vi "oax_gsExtract Order Waveform.vi"() -> ()   [LabVIEW 2017]
doc: "This VI provides Gabor order track, which can extract order from sound / vibration signal and playback on multimedia devices. This VI also provides access to Order Map.vi, which displays spectral maps, in menu bar window>> Show Order Map."
uses:
  <vilib>/addons/Sound and Vibration/Order Analysis/Ref Gabor Order Tracking/window information.ctl
  <vilib>/Analysis/1siggen.llb/Ramp Pattern by Samples.vi
  <vilib>/addons/Sound and Vibration/Order Analysis/Example Support/Demo VI/subVIs/oax_gsglobal variable.vi
  <vilib>/addons/Sound and Vibration/Order Analysis/Gabor Order Tracking/SoundVib_Gabor.lvlib
  <vilib>/Analysis/NI_AALBase.lvlib
panel:
  out "Selected File":string
  in  "Load Data":bool
  in  "user data path":path
  in  "Select Data":i32(listbox)
  in  "STOP":bool
  in  "track 3":bool
  in  "track 2":bool
  out "Speed at\nCursor (RPM)":dbl
  out "Time at\nCursor (sec)":dbl format="%.2f"
  in  "last path":path
  in  "unit":u16(ring) items=["Order", "Hz"]
  out "window information":T1={"window type"=3, "window length"=1} {"window type" items=["None"=0, "Hanning"=1, "Hamming"=2, "Blackman-Harris"=3, "Exact Blackman"=4, "Blackman"=5, "Flat Top"=6, "4 Term B-Harris"=7, "7 Term B-Harris"=8, "Low Sidelobe"=9, "Gaussian"=62]; "window length" min=0}
  out "TF Plot":u8[][](graph) caption="Time-Frequency Plot"
  out "Cursor Position":cluster{"Cursor X":dbl, "Cursor Y":dbl}={"Cursor X"=347.3140311804009, "Cursor Y"=0.0} {"Cursor Y" format="%.2f"; "Cursor X" format="%.2f"}
  in  "Play Sound":T2(ring)
  in  "Order List":i32[](listbox)
  out "Spectrum":cluster{dbl[], "X":dbl[]}(graph)
  out "mask":bool[][](array[boolean])
  in  "Bandwidth":dbl(slide)=0.5 min=0.0 scale=0.0..1.0 scale format="%.2f"
  in  "track":bool
  out "X":dbl[](array[numeric]) format="%.2f"
  in  "Selected Order":dbl min=0.0 step=0.10000000149011612 format="%.1f"
  out "Window \nLength":i32
  out "Status":string="Waiting..."
  out "Sample \nRate (Hz)":dbl
  out "S&V plot":dbl[][](graph)
  # "Narrow"
  # "Wide"
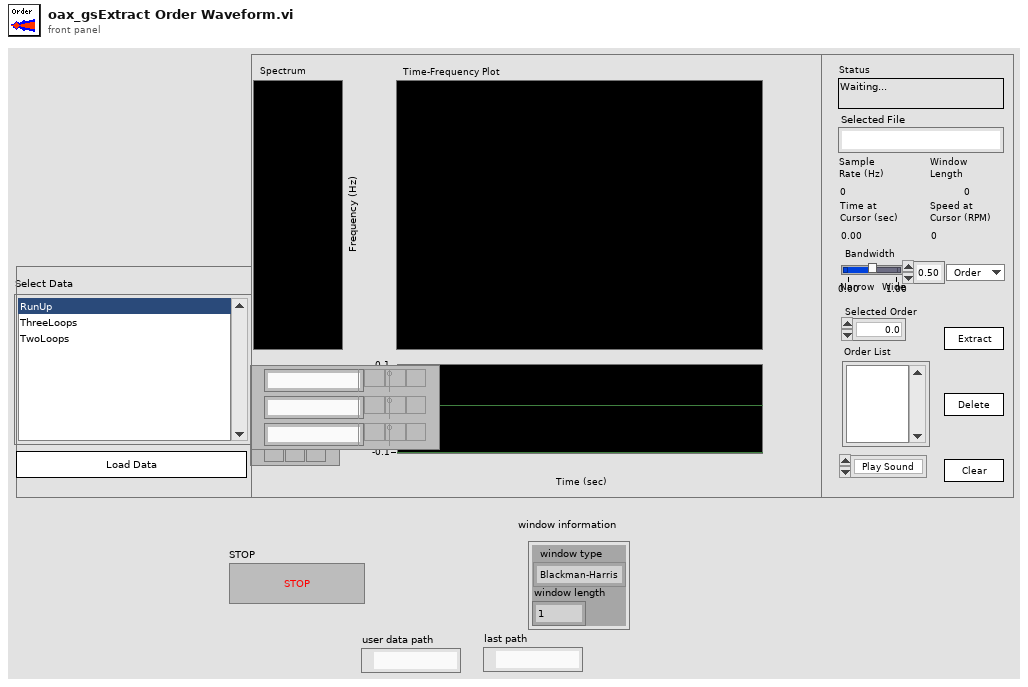
[diagram p1: front panel]
types:
  T1 = typedef "SoundVib_Gabor.lvlib/window information.ctl" = cluster{"window type":u32, "window length":i32}
  T2 = enum16{"Play Sound", "Original Signal", "Selected Orders", "Without Orders"}
  T3 = enum16{"Play Sound", "Original Samples", "Selected Orders", "Without Orders"}
  T4 = typedef "LVPointDoubleTypeDef.ctl" = cluster{"Cursor X":dbl, "Cursor Y":dbl}
  T5 = typedef "LVRangeTypeDef.ctl" = cluster{"Minimum":dbl, "Maximum":dbl, "Increment":dbl, "Minor Increment":dbl, "Start":dbl}
  T6 = cluster{"Selected Order":dbl, "Bandwidth":dbl, "unit":u16}
  T7 = typedef "SoundVib_Gabor.lvlib/GT RefNum.ctl" = refnum<k1>
  T8 = typedef "SoundVib_TachProcess.lvlib/speed profile.ctl" = cluster{"time [s]":dbl[], "speed [RPM]":dbl[]}
  T9 = cluster{"quality":enum16{"mono", "stereo"}, u32, "bits/sample":enum16{"8 bit", "16 bit"}}
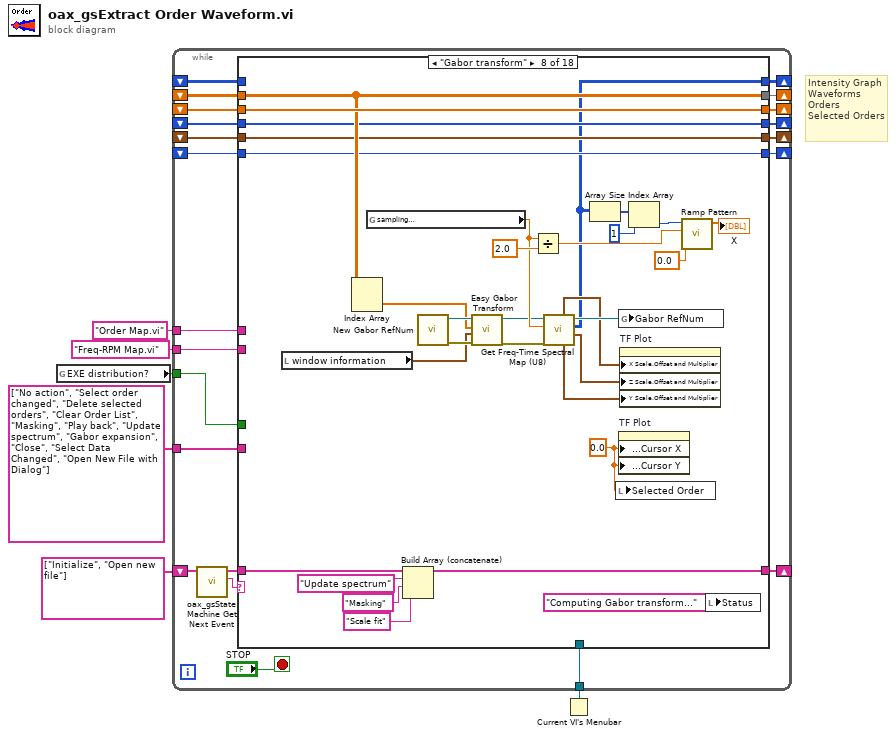
[diagram p0: block diagram]
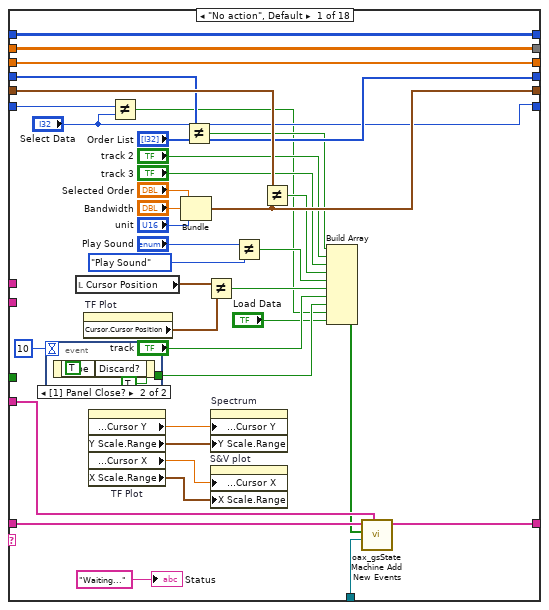
[diagram p2: hidden frame]
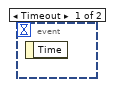
[diagram p3: hidden frame]
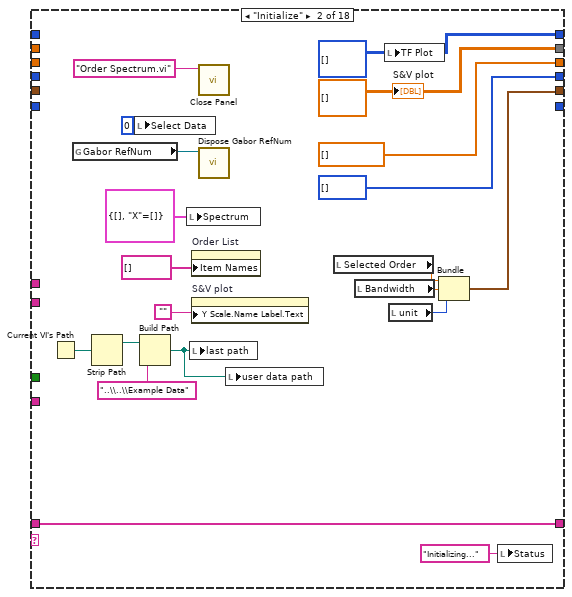
[diagram p4: hidden frame]
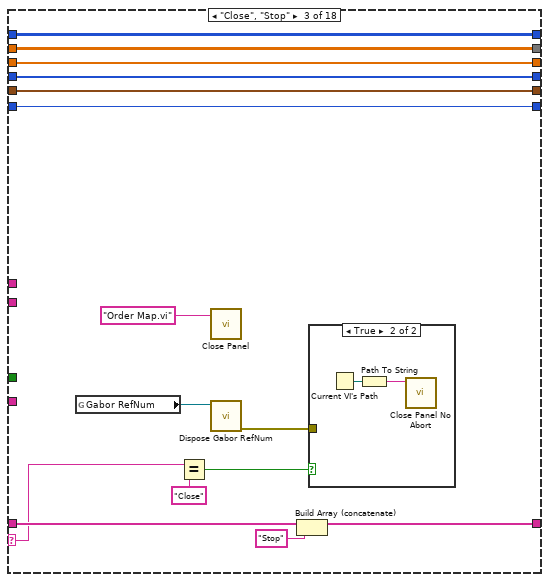
[diagram p5: hidden frame]
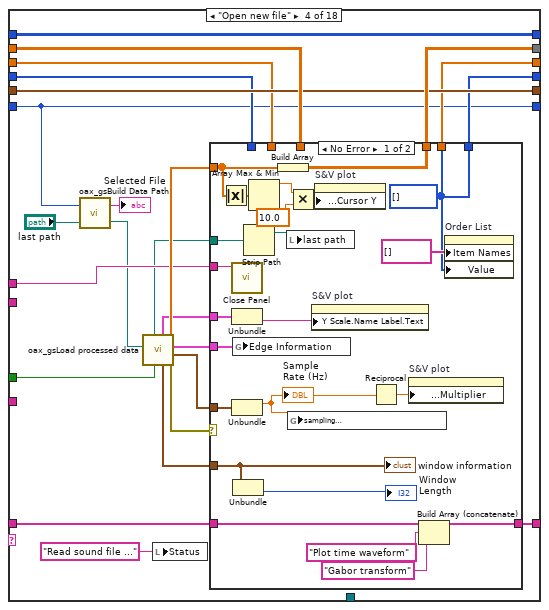
[diagram p7: hidden frame]
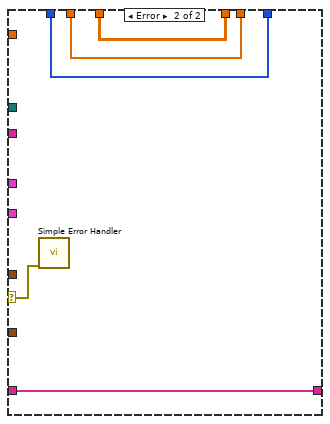
[diagram p8: hidden frame]
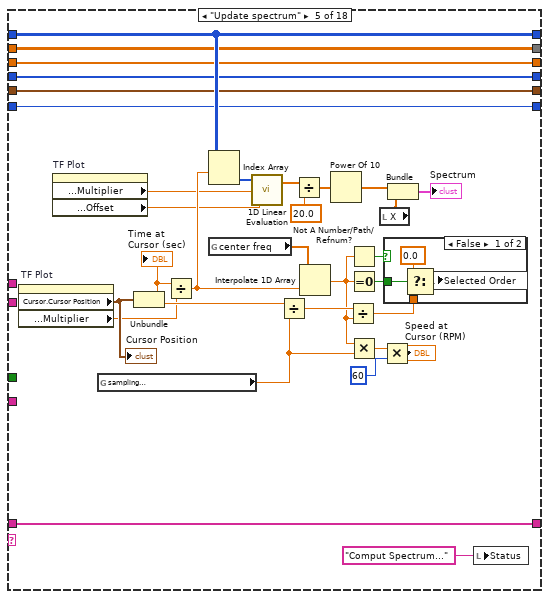
[diagram p9: hidden frame]
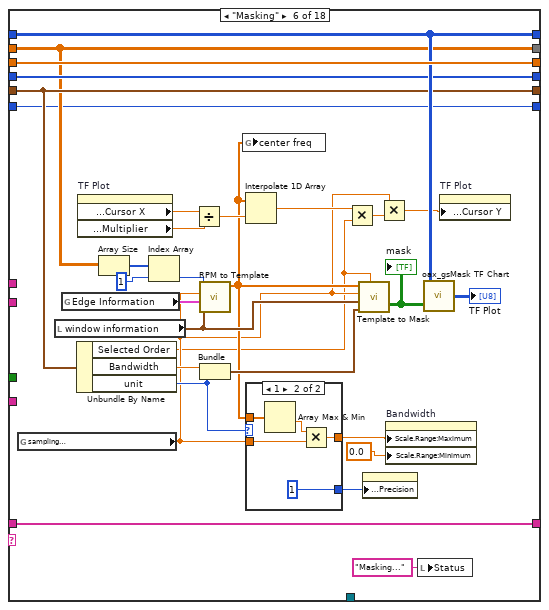
[diagram p11: hidden frame]
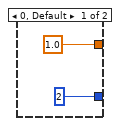
[diagram p12: hidden frame]
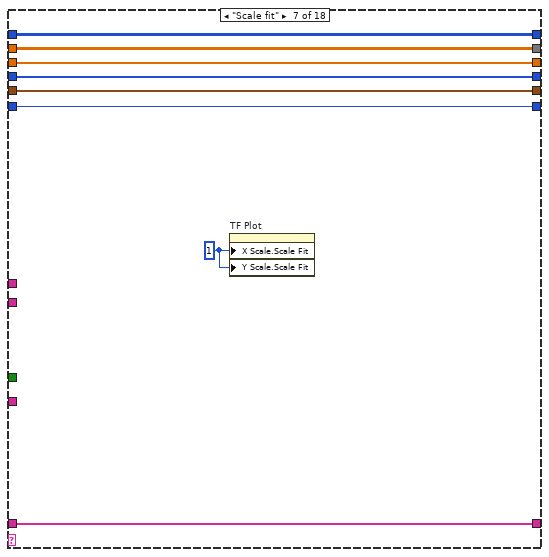
[diagram p13: hidden frame]
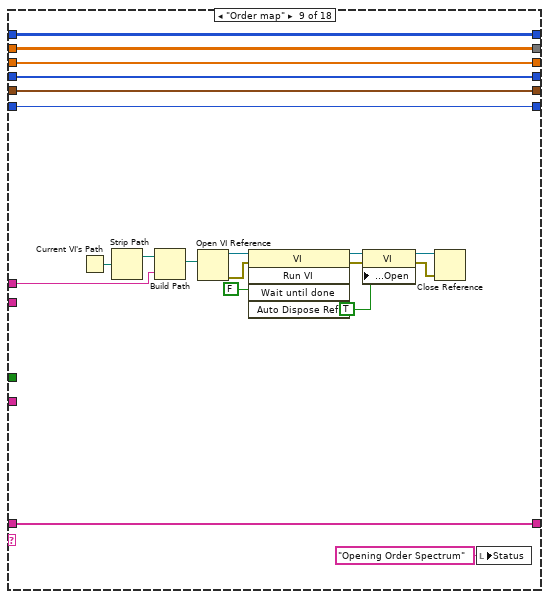
[diagram p14: hidden frame]
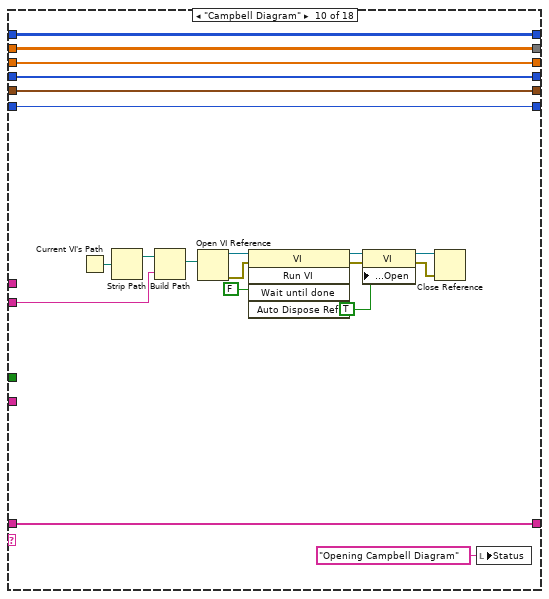
[diagram p15: hidden frame]
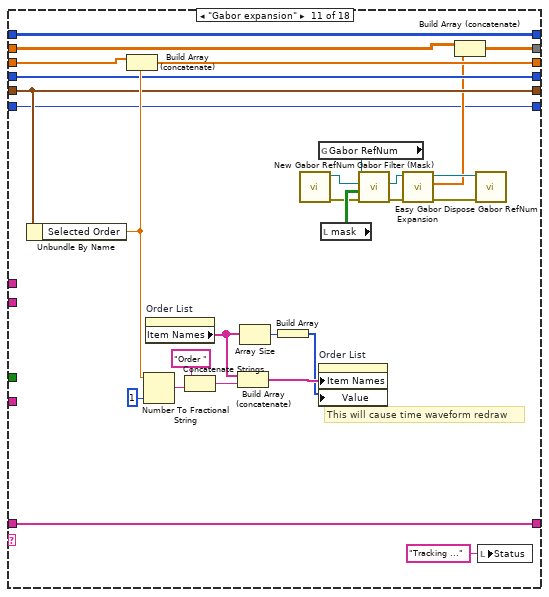
[diagram p16: hidden frame]
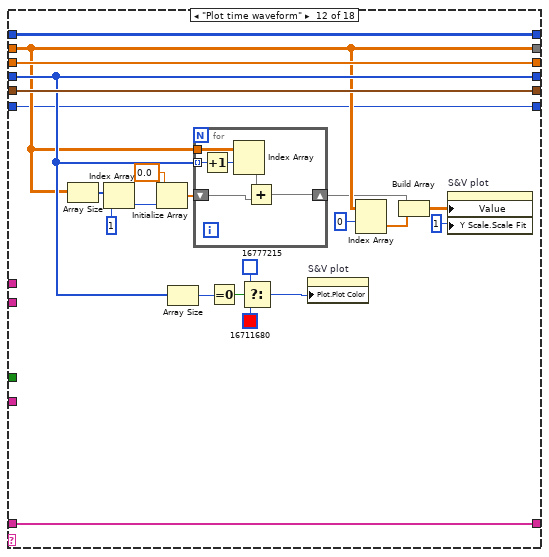
[diagram p17: hidden frame]
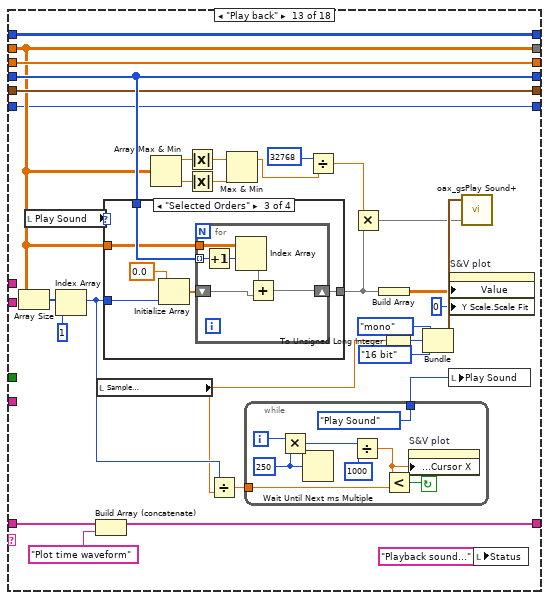
[diagram p18: hidden frame]
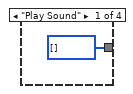
[diagram p19: hidden frame]
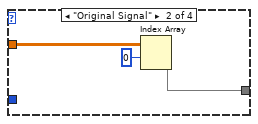
[diagram p20: hidden frame]
diagram:
  # "Intensity Graph\nWaveforms\nOrders\nSelected Orders"
  n1 = global read "oax_gsglobal variable.vi" "EXE distribution?"() -> (w2:bool)
  n2 = Current VI's Menubar() -> (w4:refnum<k9>)
  n3 = while {
    tunnel: "Freq-RPM Map.vi" ("VI name") -> [w10]
    tunnel: w2 -> [w11]
    tunnel: "Order Map.vi" ("VI name") -> [w12]
    shift-left: _ -> [w14]
    shift-right: [w13] -> _
    shift-left: _ -> [w15]
    shift-right: [w16] -> _
    tunnel: w4 -> [w17]
    tunnel: string[] ["No action", "Select order changed", "Delete selected orders", "Clear Order List", "Masking", "Play back", "Update spectrum", "Gabor expansion", "Close", "Select Data Changed", "Open New File with Dialog"] ("Event Queue Out") -> [w19]
    shift-left: string[] ["Initialize", "Open new file"] ("Event Queue Out") -> [w22]
    shift-right: [w20] -> _
    shift-left: _ -> [w23]
    shift-right: [w25] -> _
    shift-left: _ -> [w24]
    shift-right: [w26] -> _
    shift-left: _ -> [w27]
    shift-right: [w28] -> _
    shift-right: [w8] -> _
    shift-left: _ -> [w7]
    stop <- "STOP" stop-if-true
    n4 = call <vilib>:"oax_gsState Machine Get Next Event.vi"("event queue in"=w22) -> ("next event"=w18:string, "event queue out"=w21:string[])  [unwired: 5 in]
    n5 = case shown="\"Gabor transform\"" w18 {
      selector: w18 -> [_ _ w94 _ _ _ _ _ _ _ _ _ _ _ _ _ _ _]
      tunnel: [w65 w84 w102 w128 w188 w220 w234 w239 w288 w308 w333 w358 w396 w445 w458 w479 w488 w510] -> w28
      tunnel: w27 -> [w65 _ w102 w128 w188 w220 w234 _ w288 w308 w333 w358 w396 w445 w458 w479 w488 w510]
      tunnel: [w64 w76 w101 w125 w187 w213 w233 w258 w287 w307 w331 w342 w373 w439 w449 w478 w487 w507] -> w26
      tunnel: [w63 dbl[] [] w100 w111 w186 w222 w237 w260 w286 w306 w323 w345 w395 w434 w447 w477 w486 w493] -> w25
      tunnel: w24 -> [w64 _ w101 w124 w187 w213 w233 w258 w287 w307 w332 w342 w373 w440 w452 w478 w487 w506]
      tunnel: w23 -> [w63 _ w100 w113 w186 w222 w237 w260 w286 w306 w329 w345 w395 _ w448 w477 w486 w495]
      tunnel: w21 -> [w62 w81 w97 w121 w185 w201 w231 w255 w284 w304 w310 w352 w389 w444 w455 w473 w483 w503]
      tunnel: [w61 w81 w90 w122 w185 w201 w231 w254 w284 w304 w310 w352 w387 w441 w454 w472 w481 w504] -> w20
      tunnel: w19 -> [w60 _ _ _ _ _ _ _ _ _ _ _ _ _ _ _ _ _]
      tunnel: w17 -> [w58 _ _ _ _ _ _ _ _ _ _ _ _ _ _ _ _ _]
      tunnel: [w57 w77 w98 w120 w182 w216 w236 w249 w281 w301 w315 w351 w377 w438 w457 w475 w484 w502] -> w16
      tunnel: w15 -> [w56 _ w98 w120 w182 w216 w236 w249 w281 w301 w315 w351 w377 w438 w457 w475 w484 w502]
      tunnel: w14 -> [w37 _ w99 w112 w183 w215 w235 w250 w282 w302 w316 w343 w385 w437 w451 w476 w485 w494]
      tunnel: ["Order List" i32[] [] ("Order List") w99 w110 w183 w215 w235 w250 w282 w302 w316 w343 w385 w437 i32[] [] ("Order List") w476 w485 w492] -> w13
      tunnel: w12 -> [_ _ _ w115 _ _ _ _ w270 _ _ _ _ _ _ _ _ w497]
      tunnel: w11 -> [_ _ _ w109 _ _ _ _ _ _ _ _ _ _ _ _ _ w491]
      tunnel: w10 -> [_ _ _ _ _ _ _ _ _ w290 _ _ _ _ _ _ _ _]
      tunnel: ["Select Data" _ w88 w107 w157 w193 w230 w240 w269 w289 w309 w337 w365 w432 w446 w471 w480 w490] -> w8
      tunnel: w7 -> [w32 _ w88 w107 w157 w193 w230 w240 w269 w289 w309 w337 w365 w432 w446 w471 w480 w490]
      frame "No action", Default {
        n6 = event shown="[1] Panel Close?" {
          selector: _ -> [_ _]
          dyn-events: _ -> [_ _]
          timeout: 10 -> [_ _]
          tunnel: [_ TRUE] -> w33
          event Timeout {
            n7 = event-data() -> ()  [unwired: 1 in, 1 out]
          }
          event Panel Close? {
            n8 = event-data() -> ()  [unwired: 1 in, 1 out]
            n9 = event-data("Discard?"=TRUE) -> ()  [unwired: 1 in, 1 out]
          }
        }
        n10 = local read "Cursor Position"() -> (w54:cluster{"Cursor X":dbl, "Cursor Y":dbl})
        n11 = property on="TF Plot" class="IntGraph (strict)"() -> ("Cursor.Cursor Position"=w53:T4)  [unwired: 2 in, 2 out]
        n12 = property on="TF Plot" class="IntGraph (strict)"() -> ("Cursor.Cursor Position:Cursor Y"=w50:dbl, "Y Scale.Range"=w51:T5, "Cursor.Cursor Position:Cursor X"=w40:dbl, "X Scale.Range"=w41:T5)  [unwired: 2 in, 2 out]
        n13 = Not Equal?(x=w32, y="Select Data") -> (x != y?=w30:bool)
        n14 = Bundle("Selected Order"="Selected Order", "Bandwidth"="Bandwidth", "unit"="unit") -> (w57:T6)  [unwired: 1 in]
        n15 = Not Equal?(x=w37, y="Order List") -> (x != y?=w35:bool)
        n16 = Not Equal?(x=w54, y=w53) -> (x != y?=w46:bool)
        n17 = property on="Spectrum" class="XYGraph (strict)"("Cursor.Cursor Position:Cursor Y"=w50, "Y Scale.Range"=w51) -> ()  [unwired: 2 in, 2 out]
        n18 = property on="S&V plot" class="WFGraph (strict)"("Cursor.Cursor Position:Cursor X"=w40, "X Scale.Range"=w41) -> ()  [unwired: 2 in, 2 out]
        n19 = Not Equal?(x="Play Sound", y=T3."Play Sound" ("play sound")) -> (x != y?=w43:bool)
        n20 = Not Equal?(x=w56, y=w57) -> (x != y?=w47:bool)
        n21 = Build Array(w35, "track 2", "track 3", w47, w43, w46, "track", w33, w30, "Load Data") -> (w55:bool[])
        n22 = call <vilib>:"oax_gsState Machine Add New Events.vi"("Event Names"=w60, "Menu Refnum"=w58, "New Events"=w55, "Event Queue In"=w62) -> ("Event Queue Out"=w61:string[])  [unwired: 7 in]
        "Status" <- "Waiting..." ("status")
      }
      frame "Initialize" {
        w76 = dbl[][] []
        w84 = u8[][] [] ("graph [U8]")
        n23 = Current VI's Path() -> (path=w74:path)
        n24 = global read "oax_gsglobal variable.vi" "Gabor RefNum"() -> (w85:T7)
        n25 = Strip Path(path=w74) -> (stripped path=w73:path)  [unwired: 1 out]
        n26 = local write "Select Data"(0 ("Select Data")) -> ()
        n27 = Build Path(base path=w73, name or relative path="..\\..\\Example Data") -> (appended path=w69:path)
        n28 = local write "Spectrum"(cluster{dbl[], "X":dbl[]} {[], "X"=[]} ("Instantaneous\nSpectrum")) -> ()
        n29 = local write "last path"(w69) -> ()
        n30 = property on="Order List" class="LstBox (strict)"("Item Names"=string[] [] ("Write Attribute")) -> ()  [unwired: 2 in, 2 out]
        n31 = property on="S&V plot" class="WFGraph (strict)"("Y Scale.Name Label.Text"="") -> ()  [unwired: 2 in, 2 out]
        n32 = call <vilib>:"Close Panel.vi"("VI name"="Order Spectrum.vi") -> ()  [unwired: 10 in, 1 out]
        n33 = call <vilib>:"Dispose Gabor RefNum.vi"("RefNum in"=w85) -> ()  [unwired: 7 in, 1 out]
        n34 = local write "user data path"(w69) -> ()
        n35 = local read "Selected Order"() -> (w68:dbl)
        n36 = local read "Bandwidth"() -> (w78:dbl)
        n37 = local write "TF Plot"(w84) -> ()
        n38 = local read "unit"() -> (w75:u16)
        n39 = Bundle("Selected Order"=w68, "Bandwidth"=w78, "unit"=w75) -> (w77:T6)  [unwired: 1 in]
        n40 = local write "Status"("Initializing..." ("status")) -> ()
        "S&V plot" <- w76
      }
      frame "Close", "Stop" {
        n41 = global read "oax_gsglobal variable.vi" "Gabor RefNum"() -> (w96:T7)
        n42 = Equal?(x=w94, y="Close") -> (x = y?=w92:bool)
        n43 = call <vilib>:"Close Panel.vi"("VI name"="Order Map.vi") -> ()  [unwired: 10 in, 1 out]
        n44 = call <vilib>:"Dispose Gabor RefNum.vi"("RefNum in"=w96) -> ("error out"=w91:errorcluster)  [unwired: 7 in]
        n45 = Build Array (concatenate)(w97, "Stop") -> (w90:string[])
        n46 = case shown="True" w92 {
          tunnel: w91 -> [_ _]
          frame False {
          }
          frame True {
            n47 = Current VI's Path() -> (path=w104:path)
            n48 = Path To String(path=w104) -> (string=w103:string)
            n49 = call <vilib>:"Close Panel No Abort.vi"("VI name"=w103) -> ()  [unwired: 10 in, 1 out]
          }
        }
      }
      frame "Open new file" {
        n50 = call <vilib>:"oax_gsBuild Data Path.vi"("last path"="last path", "Select Data"=w107) -> ("file path"=w106:path, "Selected File"=→"Selected File":string)
        n51 = call <vilib>:"oax_gsLoad processed data.vi"("EXE distribution?"=w109, "start path"=w106) -> ("error out"=w126:errorcluster, "parameters"=w117:cluster{"sample rate":sgl, "pulses/rev":i32}, "speed profile"=w127:T8, "S&V samples"=w119:dbl[], "window info"=w116:T1, "lables"=w118:cluster{"tach lable":string, "S&V lable":string}, "file path out"=w114:path)  [unwired: 3 in]
        n52 = local write "Status"("Read sound file ..." ("status")) -> ()
        n53 = case shown="No Error" w126 {
          selector: w126 -> [_ w154]
          tunnel: w114 -> [w130 _]
          tunnel: w127 -> [w150 _]
          tunnel: w117 -> [w145 _]
          tunnel: w119 -> [w135 _]
          tunnel: [w148 w156] -> w125
          tunnel: w124 -> [_ w156]
          tunnel: [w147 w155] -> w122
          tunnel: w121 -> [w146 w155]
          tunnel: w118 -> [w143 _]
          tunnel: w116 -> [w139 _]
          tunnel: w115 -> [w151 _]
          tunnel: w113 -> [_ w153]
          tunnel: w112 -> [_ w152]
          tunnel: [w136 w153] -> w111
          tunnel: [w136 w152] -> w110
          frame No Error {
            w136 = i32[] [] ("Order List")
            n54 = Absolute Value(x=w135) -> (abs(x)=w134:dbl[])
            n55 = call <vilib>:"Close Panel.vi"("VI name"=w151) -> ()  [unwired: 10 in, 1 out]
            n56 = Unbundle(w143) -> ("S&V lable"=w142:string)  [unwired: 1 out]
            n57 = Unbundle(w145) -> ("sample rate"=w144:sgl)  [unwired: 1 out]
            "Sample \nRate (Hz)" <- w144
            n58 = global write "oax_gsglobal variable.vi" "Edge Information"(w150) -> ()
            n59 = Unbundle(w139) -> ("window length"=→"Window \nLength":i32)  [unwired: 1 out]
            n60 = Strip Path(path=w130) -> (stripped path=w129:path)  [unwired: 1 out]
            n61 = Array Max & Min(array=w134) -> (max value=w133:dbl)  [unwired: 3 out]
            n62 = Build Array(w135) -> (w148:dbl[][])
            n63 = local write "last path"(w129) -> ()
            n64 = Multiply(x=w133, y=10.0) -> (x*y=w131:dbl)
            n65 = global write "oax_gsglobal variable.vi" "sampling \nfrequency (Hz)"(w144) -> ()
            n66 = property on="S&V plot" class="WFGraph (strict)"("Y Scale.Name Label.Text"=w142) -> ()  [unwired: 2 in, 2 out]
            n67 = property on="S&V plot" class="WFGraph (strict)"("Cursor.Cursor Position:Cursor Y"=w131) -> ()  [unwired: 2 in, 2 out]
            n68 = Reciprocal(x=w144) -> (1/x=w149:sgl)
            n69 = property on="S&V plot" class="WFGraph (strict)"("X Scale.Offset and Multiplier:Multiplier"=w149) -> ()  [unwired: 2 in, 2 out]
            n70 = Build Array (concatenate)(w146, "Plot time waveform" ("status"), "Gabor transform" ("status")) -> (w147:string[])
            n71 = property on="Order List" class="LstBox (strict)"("Item Names"=string[] [], "Value"=w136) -> ()  [unwired: 2 in, 2 out]
            "window information" <- w139
          }
          frame Error {
            n72 = call <vilib>:"Simple Error Handler.vi"("error in (no error)"=w154) -> ()  [unwired: 4 in, 5 out]
          }
        }
      }
      frame "Update spectrum" {
        n73 = property on="TF Plot" class="IntGraph (strict)"() -> ("Cursor.Cursor Position"=w176:T4, "X Scale.Offset and Multiplier:Multiplier"=w173:dbl)  [unwired: 2 in, 2 out]
        "Cursor Position" <- w176
        n74 = property on="TF Plot" class="IntGraph (strict)"() -> ("Z Scale.Offset and Multiplier:Multiplier"=w168:dbl, "Z Scale.Offset and Multiplier:Offset"=w167:dbl)  [unwired: 2 in, 2 out]
        n75 = global read "oax_gsglobal variable.vi" "sampling \nfrequency (Hz)"() -> (w160:dbl)
        n76 = Unbundle(w176) -> ("Cursor X"=w162:dbl, "Cursor Y"=w175:dbl)
        "Time at\nCursor (sec)" <- w162
        n77 = Divide(x=w162, y=w173) -> (x/y=w174:dbl)
        n78 = Index Array(array=w188, index (row)=w174) -> (element=w172:u8[])  [unwired: 1 in]
        n79 = global read "oax_gsglobal variable.vi" "center freq"() -> (w166:dbl[])
        n80 = call <vilib>:"1D Linear Evaluation.vi"("offset"=w167, "scale"=w168, "X"=w172) -> ("Y[i]=X[i]*a+b"=w171:dbl[])  [unwired: 1 out]
        n81 = Divide(x=w175, y=w160) -> (x/y=w178:dbl)
        n82 = Divide(x=w171, y=20.0 ("Write Attribute")) -> (x/y=w170:dbl[])
        n83 = Interpolate 1D Array(1:w174, 2:w166) -> (0:w165:dbl)
        n84 = Power Of 10(x=w170) -> (10^x=w179:dbl[])
        n85 = Divide(x=w178, y=w165) -> (x/y=w177:dbl)
        n86 = Not A Number/Path/Refnum?(number/path/refnum=w165) -> (NaN/Path/Refnum?=w158:bool)
        n87 = Equal To 0?(x=w165) -> (x = 0?=w159:bool)
        n88 = Multiply(x=w165, y=w160) -> (x*y=w161:dbl)
        n89 = local read "X"() -> (w180:dbl[])
        n90 = Multiply(x=w161, y=60) -> (x*y=→"Speed at\nCursor (RPM)":dbl)
        n91 = case shown="False" w158 {
          tunnel: w177 -> [w192 _]
          tunnel: w159 -> [w189 _]
          frame False {
            n92 = Select(t=0.0, s=w189, f=w192) -> (s? t:f=w190:dbl)
            n93 = local write "Selected Order"(w190) -> ()
          }
          frame True {
          }
        }
        n94 = Bundle(w179, "X"=w180) -> (→"Spectrum":cluster{dbl[], "X":dbl[]})  [unwired: 1 in]
        n95 = local write "Status"("Comput Spectrum..." ("status")) -> ()
      }
      frame "Masking" {
        n96 = global read "oax_gsglobal variable.vi" "sampling \nfrequency (Hz)"() -> (w199:dbl)
        n97 = local read "window information"() -> (w208:T1)
        n98 = global read "oax_gsglobal variable.vi" "Edge Information"() -> (w214:T8)
        n99 = Unbundle By Name(w216) -> ("Selected Order"=w198:dbl, "Bandwidth"=w207:dbl, "unit"=w206:u16)
        n100 = property on="TF Plot" class="IntGraph (strict)"() -> ("Cursor.Cursor Position:Cursor X"=w221:dbl, "X Scale.Offset and Multiplier:Multiplier"=w217:dbl)  [unwired: 2 in, 2 out]
        n101 = Array Size(array=w213) -> (size(s)=w212:i32[])
        n102 = Index Array(array=w212, index=1 ("Index")) -> (element=w211:i32)
        n103 = Divide(x=w221, y=w217) -> (x/y=w218:dbl)
        n104 = call <vilib>:"RPM to Template.vi"("window info"=w208, "speed profile"=w214, "sampling frequency [Hz]"=w199, "signal length"=w211) -> ("Gabor template"=w204:dbl[])  [unwired: 6 in, 1 out]
        n105 = Bundle("Bandwidth"=w207, "unit"=w206) -> (w205:cluster{"Bandwidth":dbl, "unit":u16})  [unwired: 1 in]
        n106 = global write "oax_gsglobal variable.vi" "center freq"(w204) -> ()
        n107 = Interpolate 1D Array(1:w218, 2:w204) -> (0:w210:dbl)
        n108 = case shown="1" w206 {
          tunnel: w204 -> [_ w229]
          tunnel: w199 -> [_ w227]
          tunnel: [1.0 w226] -> w203
          tunnel: [u8 2 u8 1] -> w202
          frame 0, Default {
          }
          frame 1 {
            n109 = Array Max & Min(array=w229) -> (min value=w228:dbl)  [unwired: 3 out]
            n110 = Multiply(x=w228, y=w227) -> (x*y=w226:dbl)
          }
        }
        n111 = Multiply(x=w210, y=w198) -> (x*y=w194:dbl)
        n112 = call <vilib>:"Template to Mask.vi"("order (1.0)"=w198, "bandwidth"=w205, "window info"=w208, "sampling frequency [S/s]"=w199, "Gabor template"=w204) -> ("mask array"=w196:bool[][])  [unwired: 6 in]
        "mask" <- w196
        n113 = property class="DigNum (strict)"("Format & Precision:Precision"=w202) -> ()  [unwired: 2 in, 2 out]
        n114 = Multiply(x=w199, y=w194) -> (x*y=w197:dbl)
        n115 = property on="Bandwidth" class="Slide (strict)"("Scale.Range:Maximum"=w203, "Scale.Range:Minimum"=0.0) -> ()  [unwired: 2 in, 2 out]
        n116 = local write "Status"("Masking..." ("status")) -> ()
        n117 = call <vilib>:"oax_gsMask TF Chart.vi"("Mask Array"=w196, "TF plot"=w220) -> ("TF plot Out"=→"TF Plot":u8[][])
        n118 = property on="TF Plot" class="IntGraph (strict)"("Cursor.Cursor Position:Cursor Y"=w197) -> ()  [unwired: 2 in, 2 out]
      }
      frame "Scale fit" {
        w232 = u8 1 ("X Scale.Scale Fit")
        n119 = property on="TF Plot" class="IntGraph (strict)"("X Scale.Scale Fit"=w232, "Y Scale.Scale Fit"=w232) -> ()  [unwired: 2 in, 2 out]
      }
      frame "Gabor transform" {
        w238 = 0.0 ("Cursor.Cursor Position:Cursor X")
        n120 = local read "window information"() -> (w248:T1)
        n121 = Index Array(array=w258) -> (element=w256:dbl[])  [unwired: 2 in]
        n122 = global read "oax_gsglobal variable.vi" "sampling \nfrequency (Hz)"() -> (w247:dbl)
        n123 = Build Array (concatenate)(w255, "Update spectrum" ("status"), "Masking" ("status"), "Scale fit" ("status")) -> (w254:string[])
        n124 = call <vilib>:"New Gabor RefNum.vi"() -> ("error out"=w257:errorcluster, "RefNum"=w268:T7)  [unwired: 9 in]
        n125 = call <vilib>:"Easy Gabor Transform.vi"("error in (no error)"=w257, "window info"=w248, "x[n]"=w256, "RefNum in"=w268) -> ("error out"=w267:errorcluster, "RefNum out"=w246:T7)  [unwired: 3 in, 3 out]
        n126 = Divide(x=w247, y=2.0) -> (x/y=w262:dbl)
        n127 = call <vilib>:"Get Freq-Time Spectral Map (U8).vi"("error in (no error)"=w267, "sampling frequency [Hz]"=w247, "RefNum in"=w246) -> ("quantization info"=w243:cluster{"offset":dbl, "multiplier":dbl}, "spectral map"=w239:u8[][], "RefNum out"=w259:T7, "frequency scale"=w242:cluster{"offset":dbl, "multiplier":dbl}, "time scale"=w244:cluster{"offset":dbl, "multiplier":dbl})  [unwired: 3 in, 1 out]
        n128 = Array Size(array=w239) -> (size(s)=w266:i32[])
        n129 = local write "Selected Order"(w238) -> ()
        n130 = global write "oax_gsglobal variable.vi" "Gabor RefNum"(w259) -> ()
        n131 = property on="TF Plot" class="IntGraph (strict)"("Cursor.Cursor Position:Cursor X"=w238, "Cursor.Cursor Position:Cursor Y"=w238) -> ()  [unwired: 2 in, 2 out]
        n132 = property on="TF Plot" class="IntGraph (strict)"("X Scale.Offset and Multiplier"=w244, "Z Scale.Offset and Multiplier"=w243, "Y Scale.Offset and Multiplier"=w242) -> ()  [unwired: 2 in, 2 out]
        n133 = Index Array(array=w266, index=1 ("Index")) -> (element=w264:i32)
        n134 = call-poly <vilib>:"Ramp Pattern.vi"("start"=0.0, "end"=w262, "samples"=w264) -> ("Ramp Pattern"=→"X":dbl[])  [unwired: 7 in, 1 out]
        n135 = local write "Status"("Computing Gabor transform..." ("status")) -> ()
      }
      frame "Order map" {
        n136 = Current VI's Path() -> (path=w285:path)
        n137 = Strip Path(path=w285) -> (stripped path=w280:path)  [unwired: 1 out]
        n138 = Build Path(base path=w280, name or relative path=w270) -> (appended path=w279:path)
        n139 = Open VI Reference(vi path=w279) -> (vi reference=w278:refnum<vi>, error out=w277:errorcluster)  [unwired: 5 in]
        n140 = invoke class="VI" method="Run VI"(reference=w278, error in=w277, "Wait until done"=FALSE) -> (reference out=w275:refnum<vi>, error out=w274:errorcluster)  [unwired: 2 in, 3 out]
        n141 = property class="VI"(reference=w275, error in=w274, "Front Panel Window:Open"=TRUE) -> (reference out=w271:refnum<vi>, error out=w272:errorcluster)
        n142 = Close Reference(reference=w271, error in (no error)=w272) -> ()  [unwired: 1 out]
        n143 = local write "Status"("Opening Order Spectrum" ("status")) -> ()
      }
      frame "Campbell Diagram" {
        n144 = Current VI's Path() -> (path=w305:path)
        n145 = Strip Path(path=w305) -> (stripped path=w300:path)  [unwired: 1 out]
        n146 = Build Path(base path=w300, name or relative path=w290) -> (appended path=w299:path)
        n147 = Open VI Reference(vi path=w299) -> (vi reference=w298:refnum<vi>, error out=w297:errorcluster)  [unwired: 5 in]
        n148 = invoke class="VI" method="Run VI"(reference=w298, error in=w297, "Wait until done"=FALSE) -> (reference out=w295:refnum<vi>, error out=w294:errorcluster)  [unwired: 2 in, 3 out]
        n149 = property class="VI"(reference=w295, error in=w294, "Front Panel Window:Open"=TRUE) -> (reference out=w291:refnum<vi>, error out=w292:errorcluster)
        n150 = Close Reference(reference=w291, error in (no error)=w292) -> ()  [unwired: 1 out]
        n151 = local write "Status"("Opening Campbell Diagram" ("status")) -> ()
      }
      frame "Gabor expansion" {
        # "This will cause time waveform redraw"
        n152 = Unbundle By Name(w315) -> ("Selected Order"=w317:dbl)
        n153 = Build Array (concatenate)(w329, w317) -> (w323:dbl[])
        n154 = Number To Fractional String(number=w317, precision (6)=i16 1) -> (F-format string=w327:string)  [unwired: 2 in]
        n155 = property on="Order List" class="LstBox (strict)"() -> ("Item Names"=w313:string[])  [unwired: 2 in, 2 out]
        n156 = Concatenate Strings("Order " ("Substring"), w327) -> (w324:string)
        n157 = Build Array (concatenate)(w313, w324) -> (w322:string[])
        n158 = Array Size(array=w313) -> (size(s)=w311:i32)
        n159 = Build Array(w311) -> (w312:i32[])
        n160 = call <vilib>:"New Gabor RefNum.vi"() -> ("error out"=w319:errorcluster, "RefNum"=w335:T7)  [unwired: 9 in]
        n161 = global read "oax_gsglobal variable.vi" "Gabor RefNum"() -> (w325:T7)
        n162 = property on="Order List" class="LstBox (strict)"("Item Names"=w322, "Value"=w312) -> ()  [unwired: 2 in, 2 out]
        n163 = local read "mask"() -> (w330:bool[][])
        n164 = call <vilib>:"Gabor Filter (Mask).vi"("error in (no error)"=w319, "mask array"=w330, "dest RefNum in"=w335, "src RefNum in"=w325) -> ("error out"=w320:errorcluster, "dest RefNum out"=w336:T7)  [unwired: 5 in, 1 out]
        n165 = call <vilib>:"Easy Gabor Expansion.vi"("error in (no error)"=w320, "RefNum in"=w336) -> ("error out"=w321:errorcluster, "time waveform"=w314:dbl[], "RefNum out"=w334:T7)  [unwired: 7 in]
        n166 = Build Array (concatenate)(w332, w314) -> (w331:dbl[][])
        n167 = call <vilib>:"Dispose Gabor RefNum.vi"("error in (no error)"=w321, "RefNum in"=w334) -> ()  [unwired: 6 in, 1 out]
        n168 = local write "Status"("Tracking ..." ("status")) -> ()
      }
      frame "Plot time waveform" {
        n169 = Array Size(array=w342) -> (size(s)=w348:i32[])
        n170 = Index Array(array=w348, index=1 ("Index")) -> (element=w344:i32)
        n171 = Initialize Array(0.0 ("y"), w344) -> (w341:dbl[])
        n172 = Array Size(array=w343) -> (size(s)=w353:i32)
        n173 = for {
          tunnel: w342 -> [w363]
          tunnel: w343 -> [w362] mode=indexing
          shift-right: [w361] -> w339
          shift-left: w341 -> [w360]
          n174 = Increment(x=w362) -> (x+1=w364:i32)
          n175 = Index Array(array=w363, index (row)=w364) -> (element=w359:dbl[])  [unwired: 1 in]
          n176 = Add(x=w359, y=w360) -> (x+y=w361:dbl[])
        }
        n177 = Equal To 0?(x=w353) -> (x = 0?=w354:bool)
        n178 = Select(t=u32 16777215 ("Read Attribute"), s=w354, f=u32 16711680 ("Read Attribute")) -> (s? t:f=w357:u32)
        n179 = property on="S&V plot" class="WFGraph (strict)"("Plot.Plot Color"=w357) -> ()  [unwired: 2 in, 2 out]
        n180 = Index Array(array=w342, index (row)=0) -> (element=w338:dbl[])  [unwired: 1 in]
        n181 = Build Array(w339, w338) -> (w350:dbl[][])
        n182 = property on="S&V plot" class="WFGraph (strict)"("Value"=w350, "Y Scale.Scale Fit"=u8 1) -> ()  [unwired: 2 in, 2 out]
      }
      frame "Play back" {
        n183 = Array Size(array=w373) -> (size(s)=w372:i32[])
        n184 = local read "Play Sound"() -> (w384:T2)
        n185 = Index Array(array=w372, index=1 ("Index")) -> (element=w371:i32)
        n186 = Build Array (concatenate)(w389, "Plot time waveform" ("status")) -> (w387:string[])
        n187 = local read "Sample \nRate (Hz)"() -> (w370:dbl)
        n188 = case shown="\"Selected Orders\"" w384 {
          tunnel: w385 -> [_ _ w414 w425]
          tunnel: [i16[] [] w406 w413 w424] -> w376
          tunnel: w373 -> [_ w408 w412 w423]
          tunnel: w371 -> [_ _ w409 _]
          frame "Play Sound" {
          }
          frame "Original Signal" {
            n189 = Index Array(array=w408, index (row)=0 ("Index")) -> (element=w406:dbl[])  [unwired: 1 in]
          }
          frame "Selected Orders" {
            n190 = Initialize Array(0.0 ("y"), w409) -> (w411:dbl[])
            n191 = for {
              tunnel: w412 -> [w419]
              tunnel: w414 -> [w418] mode=indexing
              shift-right: [w417] -> w413
              shift-left: w411 -> [w416]
              n192 = Increment(x=w418) -> (x+1=w420:i32)
              n193 = Index Array(array=w419, index (row)=w420) -> (element=w415:dbl[])  [unwired: 1 in]
              n194 = Add(x=w415, y=w416) -> (x+y=w417:dbl[])
            }
          }
          frame "Without Orders" {
            n195 = Index Array(array=w423, index (row)=0 ("Index")) -> (element=w421:dbl[])  [unwired: 1 in]
            n196 = for {
              tunnel: w423 -> [w430]
              tunnel: w425 -> [w429] mode=indexing
              shift-right: [w427] -> w424
              shift-left: w421 -> [w428]
              n197 = Increment(x=w429) -> (x+1=w431:i32)
              n198 = Index Array(array=w430, index (row)=w431) -> (element=w426:dbl[])  [unwired: 1 in]
              n199 = Subtract(x=w428, y=w426) -> (x-y=w427:dbl[])
            }
          }
        }
        n200 = Array Max & Min(array=w373) -> (max value=w383:dbl, min value=w382:dbl)  [unwired: 2 out]
        n201 = Absolute Value(x=w383) -> (abs(x)=w381:dbl)
        n202 = Absolute Value(x=w382) -> (abs(x)=w380:dbl)
        n203 = Divide(x=w371, y=w370) -> (x/y=w394:dbl)
        n204 = Max & Min(x=w381, y=w380) -> (max(x,y)=w378:dbl)  [unwired: 1 out]
        n205 = while {
          tunnel: [T2."Play Sound" ("play sound")] -> w369
          tunnel: w394 -> [w399]
          i -> [w403]
          stop <- w398 continue-if-true
          w402 = u32 250 ("milliseconds to wait")
          n206 = Multiply(x=w403, y=w402) -> (x*y=w404:u32)
          n207 = Wait Until Next ms Multiple(millisecond multiple=w402) -> ()  [unwired: 1 out]
          n208 = Divide(x=w404, y=u32 1000) -> (x/y=w400:dbl)
          n209 = Less?(x=w400, y=w399) -> (x < y?=w398:bool)
          n210 = property on="S&V plot" class="WFGraph (strict)"("Cursor.Cursor Position:Cursor X"=w400) -> ()  [unwired: 2 in, 2 out]
        }
        n211 = Divide(x=32768, y=w378) -> (x/y=w375:dbl)
        n212 = Multiply(x=w375, y=w376) -> (x*y=w374:dbl[])
        n213 = Build Array(w376) -> (w368:dbl[][])
        n214 = To Unsigned Long Integer(number=w370) -> (unsigned 32bit integer=w390:u32)
        n215 = Bundle("quality"=enum16{"mono", "stereo"}."mono", w390, "bits/sample"=enum16{"8 bit", "16 bit"}."16 bit") -> (w393:T9)  [unwired: 1 in]
        n216 = local write "Play Sound"(w369) -> ()
        n217 = property on="S&V plot" class="WFGraph (strict)"("Value"=w368, "Y Scale.Scale Fit"=u8 0) -> ()  [unwired: 2 in, 2 out]
        n218 = call <vilib>:"oax_gsPlay Sound+.vi"("Array"=w374, "sound format"=w393) -> ()  [unwired: 1 in]
        n219 = local write "Status"("Playback sound..." ("status")) -> ()
      }
      frame "Clear Order List" {
        n220 = Build Array (concatenate)(w444, "Plot time waveform" ("status")) -> (w441:string[])
        n221 = Array Subset(array=w440, length (row)=1 ("Index")) -> (w439:dbl[][])  [unwired: 3 in]
        n222 = property on="Order List" class="LstBox (strict)"("Item Names"=string[] [] ("Write Attribute")) -> ()  [unwired: 2 in, 2 out]
        n223 = local read "Selected Order"() -> (w433:dbl)
        n224 = Build Array (concatenate)(dbl[] [], w433) -> (w434:dbl[])
      }
      frame "Delete selected orders" {
        n225 = Array Size(array=w451) -> (size(s)=w450:i32)
        n226 = for {
          N: w450 -> [_]
          tunnel: w451 -> [w468]
          shift-right: [w469] -> w449
          shift-left: w452 -> [w470]
          shift-right: [w466] -> _
          shift-left: w450 -> [w467]
          shift-right: [w463] -> w447
          shift-left: w448 -> [w464]
          n227 = property on="Order List" class="LstBox (strict)"() -> ("Item Names"=w461:string[])  [unwired: 2 in, 2 out]
          n228 = Decrement(x=w467) -> (x-1=w466:i32)
          n229 = Index Array(array=w468, index=w466) -> (element=w459:i32)
          n230 = Increment(x=w459) -> (x+1=w465:i32)
          n231 = Delete From Array(array=w461, index=w459) -> (array with subset deleted=w460:string[])  [unwired: 1 in, 1 out]
          n232 = Delete From Array(array=w470, index (row)=w465) -> (array with subset deleted=w469:dbl[][])  [unwired: 2 in, 1 out]
          n233 = Delete From Array(array=w464, length=1, index=w459) -> (array with subset deleted=w463:dbl[])  [unwired: 1 out]
          n234 = property on="Order List" class="LstBox (strict)"("Item Names"=w460) -> ()  [unwired: 2 in, 2 out]
        }
        n235 = Build Array (concatenate)(w455, "Plot time waveform" ("status")) -> (w454:string[])
      }
      frame "Select order changed" {
        n236 = Build Array (concatenate)(w473, "Plot time waveform" ("status")) -> (w472:string[])
      }
      frame "Select Data Changed" {
        n237 = Build Array (concatenate)(w483, string[] ["Open new file"] ("element")) -> (w481:string[])
      }
      frame "Open New File with Dialog" {
        n238 = call <vilib>:"oax_gsLoad processed data with Dialog.vi"("EXE distribution?"=w491, "start path"="user data path") -> ("error out"=w508:errorcluster, "parameters"=w499:cluster{"sample rate":sgl, "pulses/rev":i32}, "speed profile"=w509:T8, "S&V samples"=w501:dbl[], "window info"=w498:T1, "lables"=w500:cluster{"tach lable":string, "S&V lable":string}, "file path out"=w496:path)  [unwired: 3 in]
        n239 = local write "Status"("Read sound file ..." ("status")) -> ()
        n240 = case shown="No Error" w508 {
          selector: w508 -> [_ w537]
          tunnel: w496 -> [w516 _]
          tunnel: w509 -> [w533 _]
          tunnel: w499 -> [w528 _]
          tunnel: w501 -> [w521 _]
          tunnel: [w531 w539] -> w507
          tunnel: w506 -> [_ w539]
          tunnel: [w530 w538] -> w504
          tunnel: w503 -> [w529 w538]
          tunnel: w500 -> [w527 _]
          tunnel: w498 -> [w512 _]
          tunnel: w497 -> [w534 _]
          tunnel: w495 -> [_ w536]
          tunnel: w494 -> [_ w535]
          tunnel: [w522 w536] -> w493
          tunnel: [w522 w535] -> w492
          frame No Error {
            w522 = i32[] [] ("Order List")
            n241 = Absolute Value(x=w521) -> (abs(x)=w520:dbl[])
            n242 = call <vilib>:"Close Panel.vi"("VI name"=w534) -> ()  [unwired: 10 in, 1 out]
            n243 = Unbundle(w527) -> ("S&V lable"=w526:string)  [unwired: 1 out]
            n244 = Unbundle(w528) -> ("sample rate"=w513:sgl)  [unwired: 1 out]
            n245 = global write "oax_gsglobal variable.vi" "Edge Information"(w533) -> ()
            n246 = Unbundle(w512) -> ("window length"=w514:i32)  [unwired: 1 out]
            n247 = Strip Path(path=w516) -> (stripped path=w515:path, name=w511:string)
            n248 = Array Max & Min(array=w520) -> (max value=w519:dbl)  [unwired: 3 out]
            n249 = local write "Sample \nRate (Hz)"(w513) -> ()
            n250 = local write "Window \nLength"(w514) -> ()
            n251 = Build Array(w521) -> (w531:dbl[][])
            n252 = Multiply(x=w519, y=10.0) -> (x*y=w517:dbl)
            n253 = global write "oax_gsglobal variable.vi" "sampling \nfrequency (Hz)"(w513) -> ()
            n254 = local write "user data path"(w515) -> ()
            n255 = local write "Selected File"(w511) -> ()
            n256 = property on="S&V plot" class="WFGraph (strict)"("Y Scale.Name Label.Text"=w526) -> ()  [unwired: 2 in, 2 out]
            n257 = property on="S&V plot" class="WFGraph (strict)"("Cursor.Cursor Position:Cursor Y"=w517) -> ()  [unwired: 2 in, 2 out]
            n258 = local write "window information"(w512) -> ()
            n259 = Reciprocal(x=w513) -> (1/x=w532:sgl)
            n260 = property on="S&V plot" class="WFGraph (strict)"("X Scale.Offset and Multiplier:Multiplier"=w532) -> ()  [unwired: 2 in, 2 out]
            n261 = Build Array (concatenate)(w529, "Plot time waveform" ("status"), "Gabor transform" ("status")) -> (w530:string[])
            n262 = property on="Order List" class="LstBox (strict)"("Item Names"=string[] [], "Value"=w522) -> ()  [unwired: 2 in, 2 out]
          }
          frame Error {
            n263 = call <vilib>:"Simple Error Handler.vi"("error in (no error)"=w537) -> ()  [unwired: 4 in, 5 out]
          }
        }
      }
    }
  }
